vi "GetCurrentValues.vi"(8 "error in (no error)":errorcluster, 10 "OpState":variant, 11 "History":variant) -> (0 "error out":errorcluster, 2 "current values":T1[](array[typedef]))   [LabVIEW 2017, in "TestPanel.lvlib"]
uses:
  <vilib>/addons/InsightCM/Devices/Shared/Common/TestPanel/TestPanel.lvlib
  <vilib>/addons/InsightCM/MessageBus/Base/controls/TestPanelCurrentValues.ctl
  <vilib>/addons/InsightCM/MessageBus/Base/controls/KeyValuePair.ctl
  <vilib>/addons/InsightCM/MessageBus/Base/controls/TestPanelCurrentValue.ctl
  <vilib>/addons/InsightCM/MessageBus/Base/controls/TestPanelValue.ctl
  <vilib>/addons/InsightCM/MessageBus/Base/controls/TestPanelTimeSeries.ctl
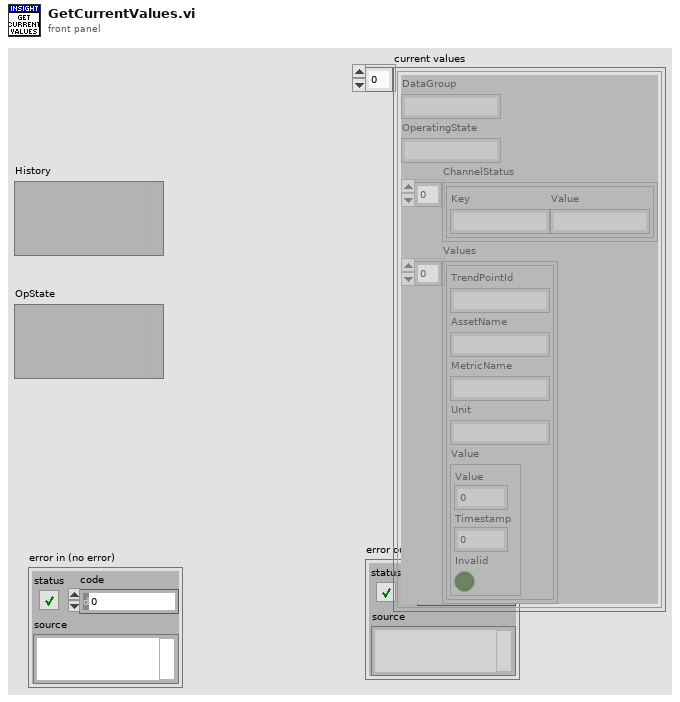
[diagram p1: front panel]
types:
  T1 = typedef "TestPanelCurrentValues.ctl" = cluster{"DataGroup":string, "OperatingState":string, "ChannelStatus":T2[], "Values":T3[]}
  T2 = typedef "KeyValuePair.ctl" = cluster{"Key":string, "Value":string}
  T3 = typedef "TestPanelCurrentValue.ctl" = cluster{"TrendPointId":string, "AssetName":string, "MetricName":string, "Unit":string, "Value":T4}
  T4 = typedef "TestPanelValue.ctl" = cluster{"Value":dbl, "Timestamp":i64, "Invalid":bool}
  T5 = typedef "TestPanelTimeSeries.ctl" = cluster{"TrendPointId":string, "AssetName":string, "MetricName":string, "Unit":string, "Values":T4[]}
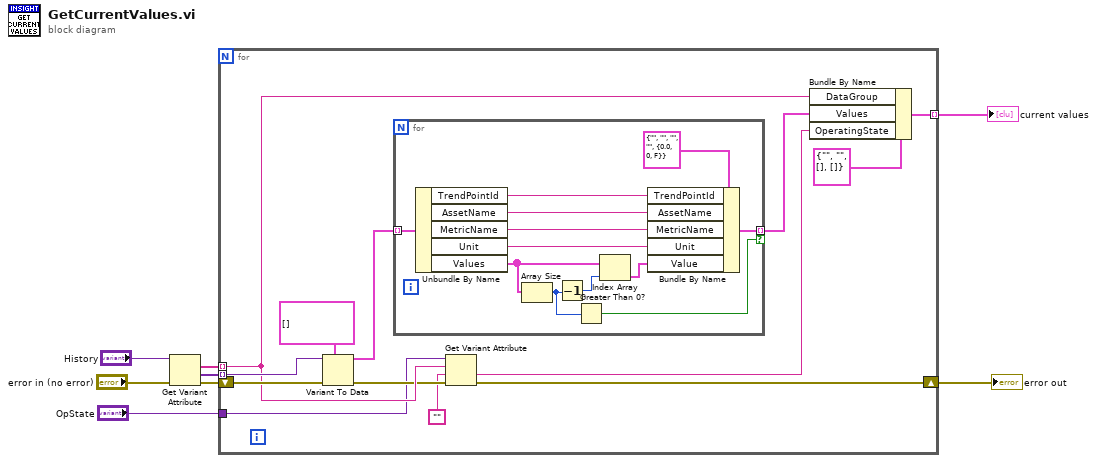
[diagram p0: block diagram]
diagram:
  n1 = Get Variant Attribute(Variant="History", error in="error in (no error)") -> (names=w5:string[], values=w6:variant[], error out=w7:errorcluster)  [unwired: 2 in, 1 out]
  n2 = for {
    shift-right: [w10] -> w2
    shift-left: w7 -> [w20]
    tunnel: w6 -> [w19] mode=indexing
    tunnel: w5 -> [w15] mode=indexing
    tunnel: "OpState" -> [w13]
    tunnel: [w9] -> w1 mode=indexing
    n3 = Variant To Data(error in=w20, type=T5[] [], Variant=w19) -> (data=w17:T5[], error out=w14:errorcluster)
    n4 = for {
      tunnel: w17 -> [w32] mode=indexing
      tunnel: [w26] -> w16 mode=indexing if=w22
      n5 = Unbundle By Name(w32) -> ("TrendPointId"=w27:string, "AssetName"=w28:string, "MetricName"=w25:string, "Unit"=w24:string, "Values"=w31:T4[])
      n6 = Array Size(array=w31) -> (size(s)=w23:i32)
      n7 = Decrement(x=w23) -> (x-1=w30:i32)
      n8 = Greater Than 0?(x=w23) -> (x > 0?=w22:bool)
      n9 = Index Array(array=w31, index=w30) -> (element=w29:T4)
      n10 = Bundle By Name(cluster=T3 {"TrendPointId"="", "AssetName"="", "MetricName"="", "Unit"="", "Value"={"Value"=0.0, "Timestamp"=0, "Invalid"=FALSE}} ("CurrentValue"), "TrendPointId"=w27, "AssetName"=w28, "MetricName"=w25, "Unit"=w24, "Value"=w29) -> (w26:T3)
    }
    n11 = Get Variant Attribute(Variant=w13, name=w15, default value (empty Variant)="", error in=w14) -> (value=w11:string, error out=w10:errorcluster)  [unwired: 2 out]
    n12 = Bundle By Name(cluster=T1 {"DataGroup"="", "OperatingState"="", "ChannelStatus"=[], "Values"=[]} ("CurrentValues"), "DataGroup"=w15, "Values"=w16, "OperatingState"=w11) -> (w9:T1)
  }
  "error out" <- w2
  "current values" <- w1
